vi "Construct SystemLog Sink.vi"(7 "LogLevel":T1=enum."Info", 11 "LogFormat":refnum<class "IStringFormat.lvclass">) -> (3 "SystemLog Sink out":refnum<class "SystemLog Sink.lvclass">)   [LabVIEW 2020, in "MVA Framework.lvlib" / "SystemLog Sink.lvclass"]
uses:
  SystemLog Sink.lvclass
  IStringFormat/IStringFormat.lvclass
  Composed Log/Types/Log Level.ctl
  Composed Log/Log Sink/Log Sink.lvclass/Log Sink.ctl
  String Log Sink/String Log Sink.lvclass/String Log Sink.ctl
  SystemLog Sink.lvclass/SystemLog Sink.ctl
  Composed Log/Log Sink/Log Sink.lvclass
  String Log Sink/String Log Sink.lvclass
  Composed Log/Composed Log.lvlib
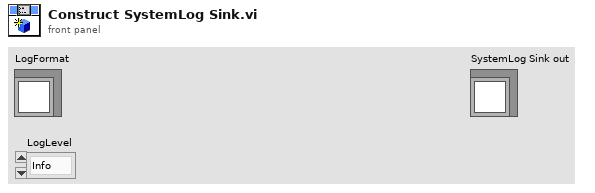
[diagram p1: front panel]
types:
  T1 = typedef "MVA Framework.lvlib/Composed Log.lvlib/Log Level.ctl" = enum16{"Debug", "Info", "Warning", "Error", "Critical"}
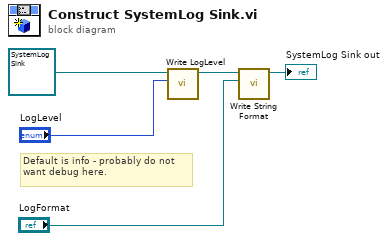
[diagram p0: block diagram]
diagram:
  # "Default is info - probably do not want debug here."
  n1 = call "Write LogLevel.vi"("LogLevel"="LogLevel", "Log Sink in"=refnum<class "SystemLog Sink.lvclass"> refnum ("SystemLog Sink in")) -> ("Log Sink out"=w3:refnum<class "SystemLog Sink.lvclass">)  [unwired: 8 in, 1 out]
  n2 = call "Write String Format.vi"("StringFormat"="LogFormat", "String Log Sink in"=w3) -> ("String Log Sink out"=→"SystemLog Sink out":refnum<class "SystemLog Sink.lvclass">)  [unwired: 8 in, 1 out]
